vi "Getting Started.vi"() -> ()   [LabVIEW 2015]
panel:
  out "Error Number":i32
  out "Error Message":string
  out "ID responce":string
  out "Address \"OK\"":string
  in  "UVP_UVL selector":bool
  out "error out":errorcluster
  out "Output Current":dbl format="%.4f"
  out "Output Voltage":dbl format="%.4f"
  in  "Output ON":bool=TRUE
  in  "OVP":dbl format="%.4f"
  in  "UVL UVP value":dbl format="%.4f"
  in  "Current Limit":dbl format="%.4f"
  in  "Voltage Limit":dbl format="%.4f"
  in  "Reset (T)":bool
  in  "Address":i16=6
  in  "Language Selector":i16(ring)=1 items=["GEN", "SCPI"]
  in  "error in":errorcluster
  in  "ID Query (T)":bool=TRUE
  in  "Baud Rate":i32(ring)=3 items=["1200", "2400", "4800", "9600", "19200", "38400", "57600", "115200"]
  in  "VISA":refnum<visa-resource-name>
  # "1. Set Propertly Communication Parameters\n2. Set Required Output Values and then  RUN"
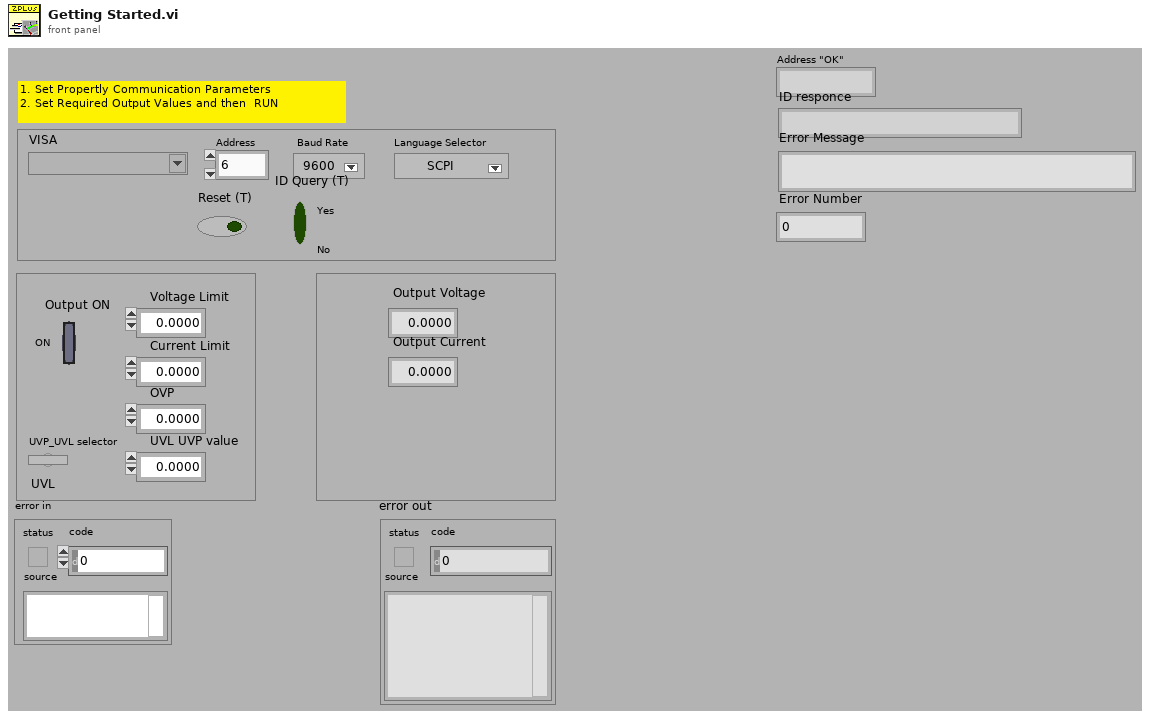
[diagram p1: front panel]
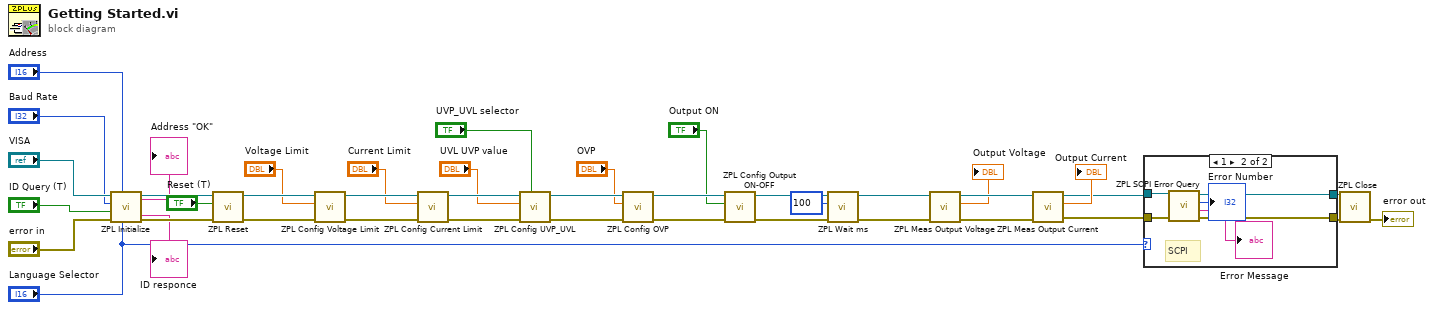
[diagram p0: block diagram]
diagram:
  n1 = call "ZPL Initialize.vi"("Language Selector"="Language Selector", "Address"="Address", "error in"="error in", "ID Query (T)"="ID Query (T)", "Baud Rate"="Baud Rate", "VISA"="VISA") -> ("error out"=w32:errorcluster, "VISA  out"=w41:refnum<visa-resource-name>, "ID responce"=→"ID responce":string, "Address \"OK\""=→"Address \"OK\"":string)  [unwired: 2 in]
  n2 = call "ZPL Reset.vi"("error"=w32, "Reset (T)"="Reset (T)", "VISA"=w41) -> ("error out"=w31:errorcluster, "VISA out"=w40:refnum<visa-resource-name>)  [unwired: 7 in]
  n3 = call "ZPL Config Voltage Limit.vi"("error"=w31, "Voltage Limit"="Voltage Limit", "VISA"=w40) -> ("error out"=w30:errorcluster, "VISA out"=w39:refnum<visa-resource-name>)  [unwired: 7 in]
  n4 = call "ZPL Config Current Limit.vi"("error"=w30, "Current Limit"="Current Limit", "VISA"=w39) -> ("error out"=w29:errorcluster, "VISA out"=w38:refnum<visa-resource-name>)  [unwired: 7 in]
  n5 = call "ZPL Config UVP_UVL.vi"("UVP_UVL selector"="UVP_UVL selector", "error"=w29, "UVL UVP value"="UVL UVP value", "VISA"=w38) -> ("error out"=w28:errorcluster, "VISA out"=w37:refnum<visa-resource-name>)  [unwired: 6 in]
  n6 = call "ZPL Config OVP.vi"("error"=w28, "OVP"="OVP", "VISA"=w37) -> ("error out"=w27:errorcluster, "VISA out"=w36:refnum<visa-resource-name>)  [unwired: 7 in]
  n7 = call "ZPL Config Output ON-OFF.vi"("error"=w27, "Output ON"="Output ON", "VISA"=w36) -> ("error out"=w26:errorcluster, "VISA out"=w35:refnum<visa-resource-name>)  [unwired: 7 in]
  n8 = call "ZPL Wait ms.vi"("error"=w26, "Delay (1 mS)"=u32 100, "VISA"=w35) -> ("error out"=w25:errorcluster, "VISA out"=w34:refnum<visa-resource-name>)  [unwired: 7 in]
  n9 = call "ZPL Meas Output Voltage.vi"("error"=w25, "VISA"=w34) -> ("error out"=w24:errorcluster, "Output Voltage"=→"Output Voltage":dbl, "VISA out"=w33:refnum<visa-resource-name>)  [unwired: 7 in]
  n10 = call "ZPL Meas Output Current.vi"("error"=w24, "VISA"=w33) -> ("error out"=w8:errorcluster, "Output Current"=→"Output Current":dbl, "VISA out"=w9:refnum<visa-resource-name>)  [unwired: 7 in]
  n11 = case shown="1" "Language Selector" {
    tunnel: w9 -> [w43 w49]
    tunnel: w8 -> [w42 w48]
    tunnel: [w43 w47] -> w7
    tunnel: [w42 w46] -> w6
    frame 0, Default {
      # "GEN"
    }
    frame 1 {
      # "SCPI"
      n12 = call "ZPL SCPI Error Query.vi"("error"=w48, "VISA"=w49) -> ("error out"=w46:errorcluster, "Error Message"=→"Error Message":string, "Error Number"=→"Error Number":i32, "VISA out"=w47:refnum<visa-resource-name>)  [unwired: 6 in]
    }
  }
  n13 = call "ZPL Close.vi"("error"=w6, "VISA name"=w7) -> ("error out"=→"error out":errorcluster)  [unwired: 7 in]
